vi "Read_Clk_Rates.vi"(8 "error in":errorcluster, 11 "VISA in":refnum<visa-resource-name>) -> (0 "error out":errorcluster, 3 "VISA out":refnum<visa-resource-name>, 4 "Clk Rates":T1)   [LabVIEW 2019]
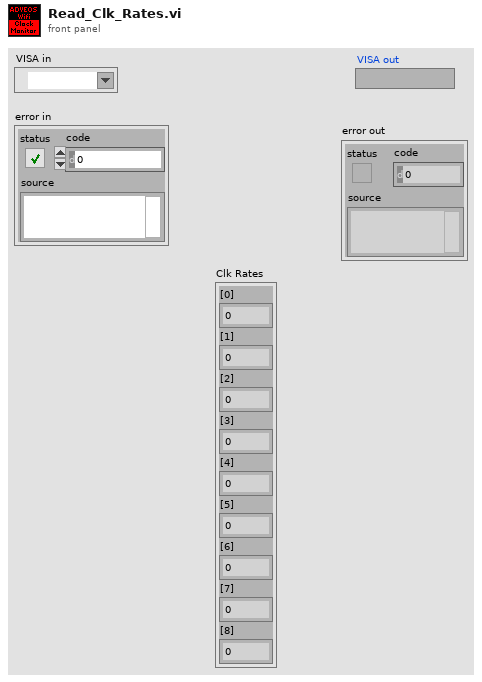
[diagram p1: front panel]
types:
  T1 = cluster{"[0]":u32, "[1]":u32, "[2]":u32, "[3]":u32, "[4]":u32, "[5]":u32, "[6]":u32, "[7]":u32, "[8]":u32}
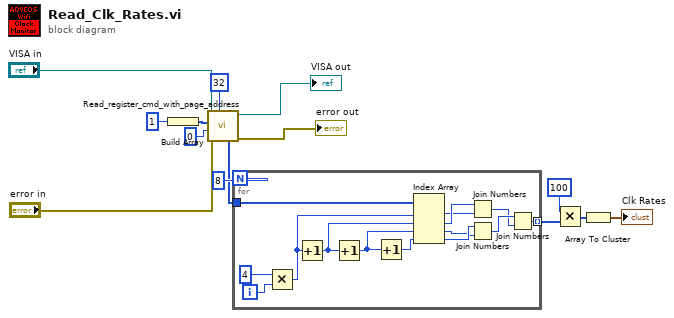
[diagram p0: block diagram]
diagram:
  n1 = Build Array(u8 1) -> (w6:u8[])
  n2 = call "Read_register_cmd_with_page_address.vi"("Words_to_read"=u16 32, "error in (no error)"="error in", "Register Address"=u8 0, "Page address"=w6, "VISA Refnum in"="VISA in") -> ("error out"=→"error out":errorcluster, "VISA Refnum out"=→"VISA out":refnum<visa-resource-name>, "RdReg Data"=w12:u8[])  [unwired: 4 in]
  n3 = for {
    N: 8 -> [_]
    tunnel: w12 -> [w28]
    tunnel: [w15] -> w14 mode=indexing
    i -> [w27]
    n4 = Multiply(x=4, y=w27) -> (x*y=w25:i32)
    n5 = Increment(x=w25) -> (x+1=w24:i32)
    n6 = Increment(x=w24) -> (x+1=w22:i32)
    n7 = Increment(x=w22) -> (x+1=w23:i32)
    n8 = Index Array(array=w28, index #1=w25, index #2=w24, index #3=w22, index #4=w23) -> (element #1=w20:u8, element #2=w21:u8, element #3=w18:u8, element #4=w19:u8)
    n9 = Join Numbers(hi=w21, lo=w20) -> ((hi.lo)=w16:u16)
    n10 = Join Numbers(hi=w19, lo=w18) -> ((hi.lo)=w17:u16)
    n11 = Join Numbers(hi=w17, lo=w16) -> ((hi.lo)=w15:u32)
  }
  n12 = Multiply(x=100, y=w14) -> (x*y=w3:u32[])
  n13 = Array To Cluster(array=w3) -> (cluster=→"Clk Rates":T1)
